vi "Add.vi"(8 "error in (no error)":errorcluster caption="错误输入（无错误）", 10 "Size 输入 2":refnum<class "Size.lvclass"> caption="DNL_LabVIEW Object in", 11 "Size 输入":refnum<class "Size.lvclass"> caption="DNL_LabVIEW Object in") -> (0 "error out":errorcluster caption="错误输出", 3 "Size 输出":refnum<class "Size.lvclass"> caption="DNL_LabVIEW Object out")   [LabVIEW 2011, in "Size.lvclass"]
uses:
  Size.lvclass
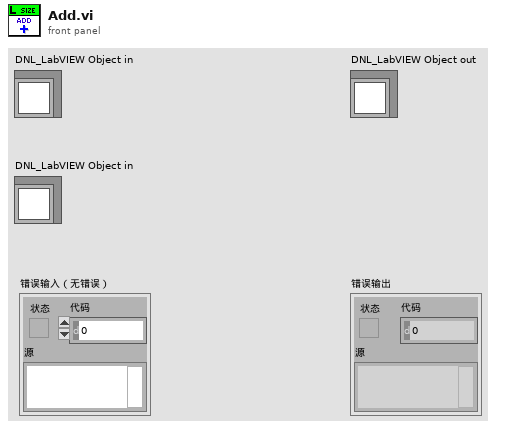
[diagram p1: front panel]
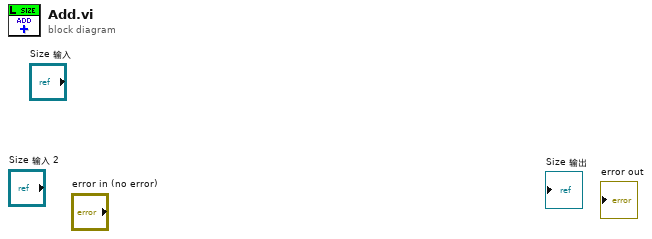
[diagram p0: block diagram]
diagram:
